vi "Compass Start I2C.vi"(8 "error in (no error)":errorcluster, 11 "Refnum in":T2) -> (0 "error out":errorcluster, 3 "FPGA Information Out":T1)   [LabVIEW 2012, in "Compass IO.lvlib"]
uses:
  Compass IO.lvlib
  FPGA_ref.ctl
  <vilib>/IEDriver/SPIandI2C/Host/I2C/I2C Host.lvlib
panel:
  in  "Address Type (7-bit)":enum16{"7-bit", "10-bit"}(ring)
  in  "Clock Rate":u32=5000
  in  "FPGA Clock (40 MHz)":u32=40000000
  in  "Port Number":u8
  in  "Address":u16=33
  # "Compass Start I2C\n---------------------\nSetup I2C address to talk with HMCxxxx compass module"
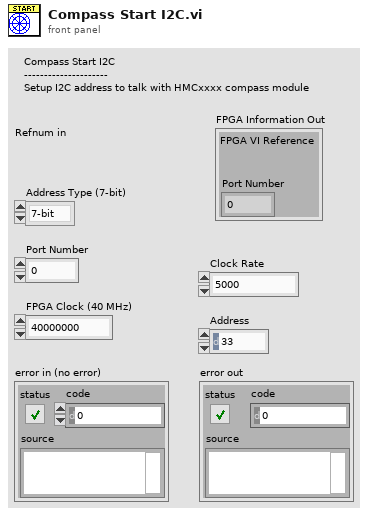
[diagram p1: front panel]
types:
  T1 = cluster{"FPGA VI Reference":refnum<k20>, "Port Number":u8}
  T2 = typedef "FPGA_ref.ctl" = refnum<k20>
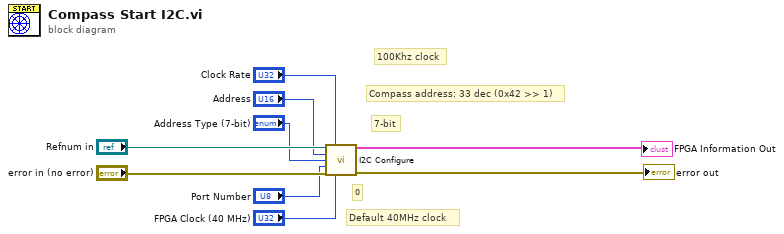
[diagram p0: block diagram]
diagram:
  # "100Khz clock"
  # "0"
  # "7-bit"
  # "Compass address: 33 dec (0x42 >> 1)"
  # "Default 40MHz clock"
  n1 = call <vilib>:"I2C Configure.vi"("FPGA VI Reference"="Refnum in", "Clock Rate"="Clock Rate", "Address"="Address", "Address Type (7-bit)"="Address Type (7-bit)", "Port Number"="Port Number", "error in (no error)"="error in (no error)", "FPGA Clock (40 MHz)"="FPGA Clock (40 MHz)") -> ("FPGA Information Out"=→"FPGA Information Out":T1, "error out"=→"error out":errorcluster)  [unwired: 7 in]
